vi "Insert Subpanel UI.vi"(2 "error in (no error)":errorcluster, 3 "Subpanel":refnum<vi>, 4 "Controller in":refnum<class "Generic Plugin.lvclass">) -> (0 "error out":errorcluster, 1 "Controller out":refnum<class "Generic Plugin.lvclass">)   [LabVIEW 2020, in "Generic Plugin.lvclass"]
doc: "Insert the Subpanel UI of the controller into the provided subpanel. The subpanel MUST have been initialized before calling this!"
uses:
  Generic Plugin.lvclass
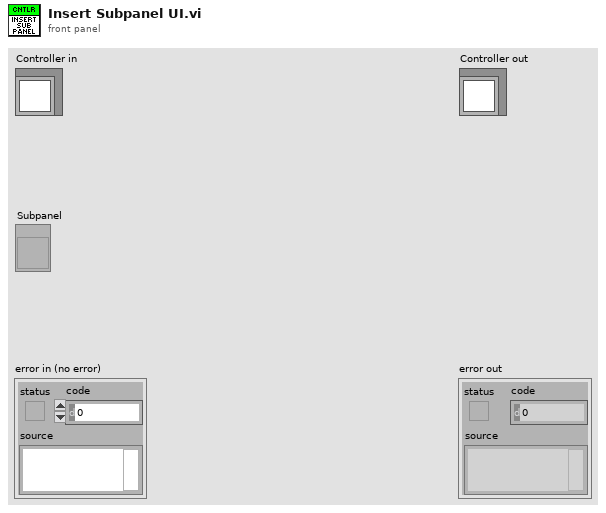
[diagram p1: front panel]
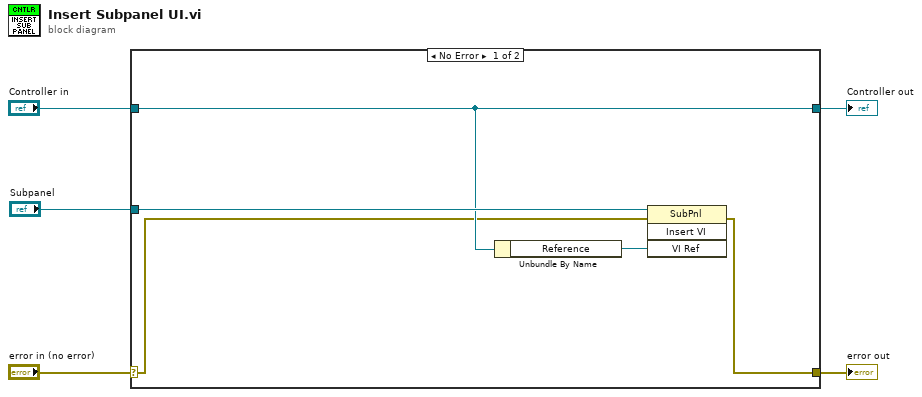
[diagram p0: block diagram]
diagram:
  n1 = case shown="No Error" "error in (no error)" {
    selector: "error in (no error)" -> [w7 w12]
    tunnel: [w10 w12] -> w4
    tunnel: [w8 w11] -> w2
    tunnel: "Controller in" -> [w8 w11]
    tunnel: "Subpanel" -> [w9 _]
    frame No Error {
      n2 = Unbundle By Name(w8) -> ("Reference"=w6:refnum<vi>)
      n3 = invoke class="SubPnl" method="Insert VI"(reference=w9, error in=w7, "VI Ref"=w6) -> (error out=w10:errorcluster)  [unwired: 1 in, 3 out]
    }
    frame Error {
    }
  }
  "error out" <- w4
  "Controller out" <- w2
